vi "ListAllReposBranches.vi"(8 "error in (no error)":errorcluster, 11 "CommandLine":string[](array[string])) -> (0 "error out":errorcluster, 2 "test details":string)   [LabVIEW 2019]
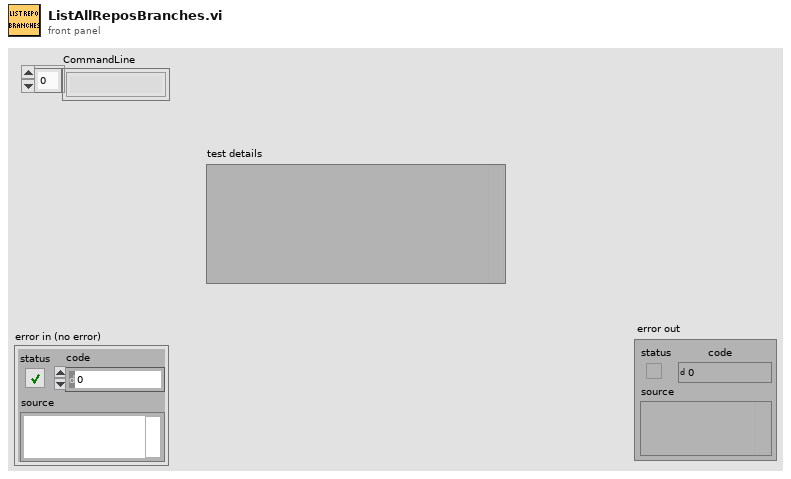
[diagram p1: front panel]
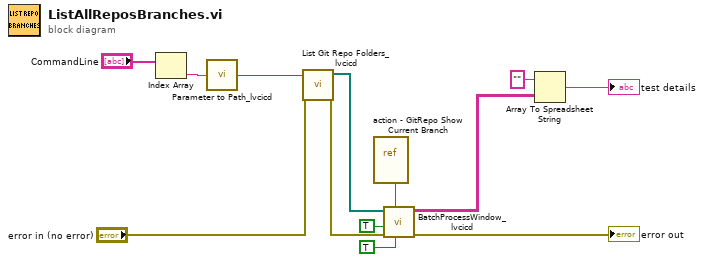
[diagram p0: block diagram]
diagram:
  n1 = Index Array(array="CommandLine") -> (element=w2:string)  [unwired: 1 in]
  n2 = call "Parameter to Path_lvcicd.vi"("String"=w2) -> ("Path"=w1:path)
  n3 = call "List Git Repo Folders_lvcicd.vi"("error in (no error)"="error in (no error)", "path"=w1) -> ("error out"=w6:errorcluster, "Repo Folders"=w12:path[])  [unwired: 8 in]
  n4 = vi-ref "action - GitRepo Show Current Branch.vi"() -> (w7:refnum<vi>)
  n5 = call "BatchProcessWindow_lvcicd.vi"("FP(T)"=TRUE, "VI Refnum"=w7, "error in (no error)"=w6, "silence mode(F)"=TRUE, "paths"=w12) -> ("error out"=→"error out":errorcluster, "Array"=w11:string[][])  [unwired: 5 in]
  n6 = Array To Spreadsheet String(array=w11, 3:"" ("format string")) -> (spreadsheet string=→"test details":string)  [unwired: 1 in]
